vi "Get Available Codecs.vi"(8 "Error In":errorcluster) -> (0 "Error Out":errorcluster, 2 "Combo Box Items":T1)   [LabVIEW 2014, in "Character Encoding Conversion.lvlib"]
doc: "Copyright (c) 2016 Sze Howe Koh\nThis code is licensed under the MIT license"
uses:
  <vilib>/Utility/miscctls.llb/LVComboBoxStrsAndValuesArrayTypeDef.ctl
  Character Encoding Conversion.lvlib
  src/LabVIEW/LQ Core/QTextCodec/QTextCodec.lvclass
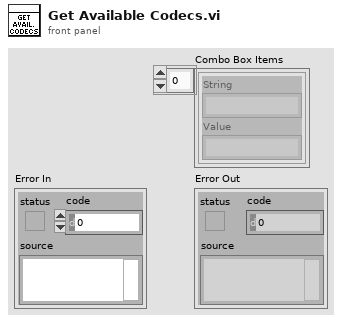
[diagram p1: front panel]
types:
  T1 = typedef "LVComboBoxStrsAndValuesArrayTypeDef.ctl" = cluster{"String":string, "Value":string}[]
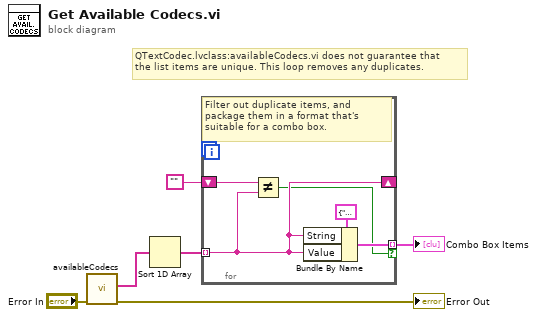
[diagram p0: block diagram]
diagram:
  # "QTextCodec.lvclass:availableCodecs.vi does not guarantee that\nthe list items are unique. This loop removes any duplicates."
  n1 = call "availableCodecs.vi"("Error In"="Error In") -> ("Error Out"=→"Error Out":errorcluster, "Value"=w6:string[])  [unwired: 9 in]
  n2 = Sort 1D Array(array=w6) -> (sorted array=w5:string[])
  n3 = for {
    tunnel: w5 -> [w9] mode=indexing
    shift-right: [w9] -> _
    shift-left: "" -> [w11]
    tunnel: [w8] -> w3 mode=indexing if=w7
    # "Filter out duplicate items, and package them in a format that's suitable for a combo box."
    n4 = Not Equal?(x=w11, y=w9) -> (x != y?=w7:bool)
    n5 = Bundle By Name(cluster=cluster{"String":string, "Value":string} {"String"="", "Value"=""}, "String"=w9, "Value"=w9) -> (w8:cluster{"String":string, "Value":string})
  }
  "Combo Box Items" <- w3
